vi "Reentrant VI Launcher.vi"   [LabVIEW 2011]
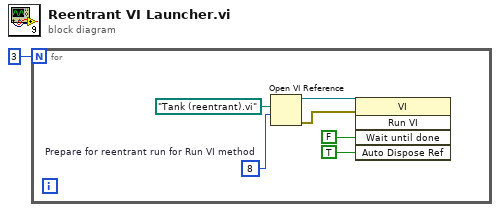
[diagram p0: block diagram]
diagram:
  n1 = for {
    N: 3 -> [_]
    w2 = 8  # Prepare for reentrant run for Run VI method
    n2 = Open VI Reference(vi path=path "Tank (reentrant).vi", options=w2) -> (vi reference=w4:refnum<vi>, error out=w3:errorcluster)  [unwired: 4 in]
    n3 = invoke class="VI" method="Run VI"(reference=w4, error in=w3, "Wait until done"=FALSE ("Wait Until Done"), "Auto Dispose Ref"=TRUE ("Auto Dispose Reference")) -> ()  [unwired: 1 in, 5 out]
  }
